vi "Destroy User Events.vi"(8 "error in (no error)":errorcluster, 11 "User Events Cluster_UI":T2) -> (0 "error out":errorcluster)   [LabVIEW 2019, in "ZenGage v3.0 UI.lvclass"]
uses:
  ZenGage v3.0 UI.lvclass
  Type Definitions/User Events UI/Optics diagnostics cluster.ctl
  <vilib>/vision/Image Controls.llb/IMAQ Image.ctl
  Type Definitions/Inspection/Result Cluster.ctl
  Type Definitions/User Events UI/LoadingBar_General_UI.ctl
  Common/Controls/Pop-up Input.ctl
  Type Definitions/JSON Read/Data initialization.ctl
  Type Definitions/JSON Read/Post select init.ctl
  Type Definitions/Diagnostics/Trigger sensor.ctl
  Type Definitions/User Events UI/UserEvents_UI.ctl
  Type Definitions/JSON Read/UI JSON read cluster.ctl
  Type Definitions/General/JSONRead.ctl
  Type Definitions/Inspection/Inspection Cluster.ctl
  Type Definitions/Diagnostics/Diagnostics(Cluster).ctl
  Type Definitions/Edit tolerance settings/Rack Selection.ctl
  <vilib>/Utility/miscctls.llb/LVPoint32TypeDef.ctl
  Type Definitions/Edit tolerance settings/Edit Tolerance Input.ctl
  Type Definitions/Edit tolerance settings/Edit Tolerance Overall Cluster.ctl
  Type Definitions/Controls and Indicators/Select a part (combobox).ctl
  Type Definitions/Controls and Indicators/EDL control references.ctl
  Type Definitions/Controls and Indicators/Diagnostics control referencs.ctl
  Type Definitions/Controls and Indicators/Inspection control references.ctl
  Type Definitions/Controls and Indicators/General_Control references.ctl
  Type Definitions/Controls and Indicators/Controls and Indicators Cluster.ctl
  Type Definitions/General/UI States(UI button enable disable).ctl
  Type Definitions/General/UIDataCluster.ctl
  Type Definitions/User Events UI/Stop slave cluster.ctl
  Type Definitions/General/Master sample references.ctl
panel:
  in  "Slave Loop":T1
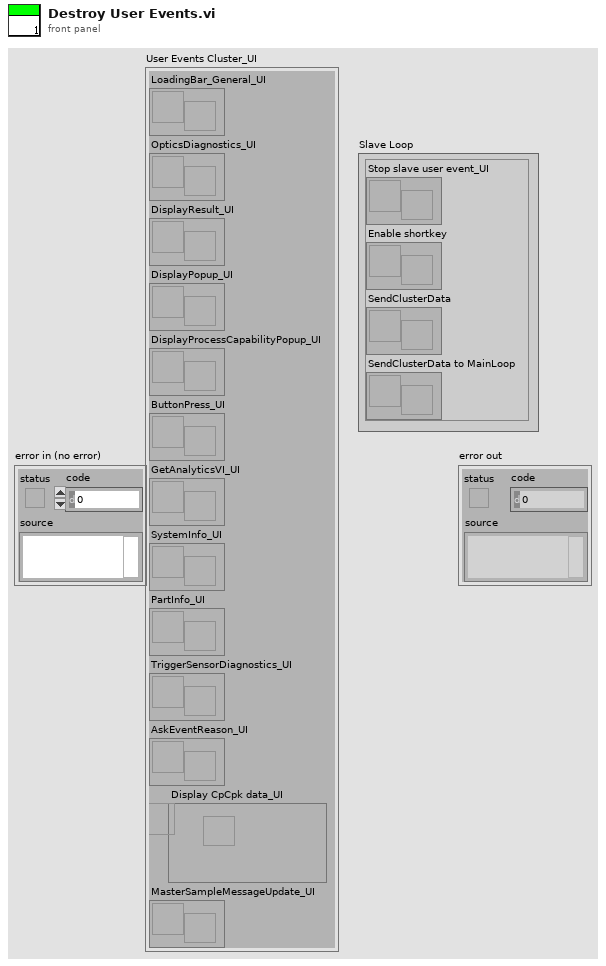
[diagram p1: front panel]
types:
  T1 = cluster{"Stop slave user event_UI":refnum<user-event>, "Enable shortkey":refnum<user-event>, "SendClusterData":refnum<user-event>, "SendClusterData to MainLoop":refnum<user-event>}
  T2 = typedef "ZenGage v3.0 UI.lvclass/UserEvents_UI.ctl" = cluster{"LoadingBar_General_UI":refnum<user-event>, "OpticsDiagnostics_UI":refnum<user-event>, "DisplayResult_UI":refnum<user-event>, "DisplayPopup_UI":refnum<user-event>, "DisplayProcessCapabilityPopup_UI":refnum<user-event>, "ButtonPress_UI":refnum<user-event>, "GetAnalyticsVI_UI":refnum<user-event>, "SystemInfo_UI":refnum<user-event>, "PartInfo_UI":refnum<user-event>, "TriggerSensorDiagnostics_UI":refnum<user-event>, "AskEventReason_UI":refnum<user-event>, "Display CpCpk data_UI":refnum<user-event>, "MasterSampleMessageUpdate_UI":refnum<user-event>}
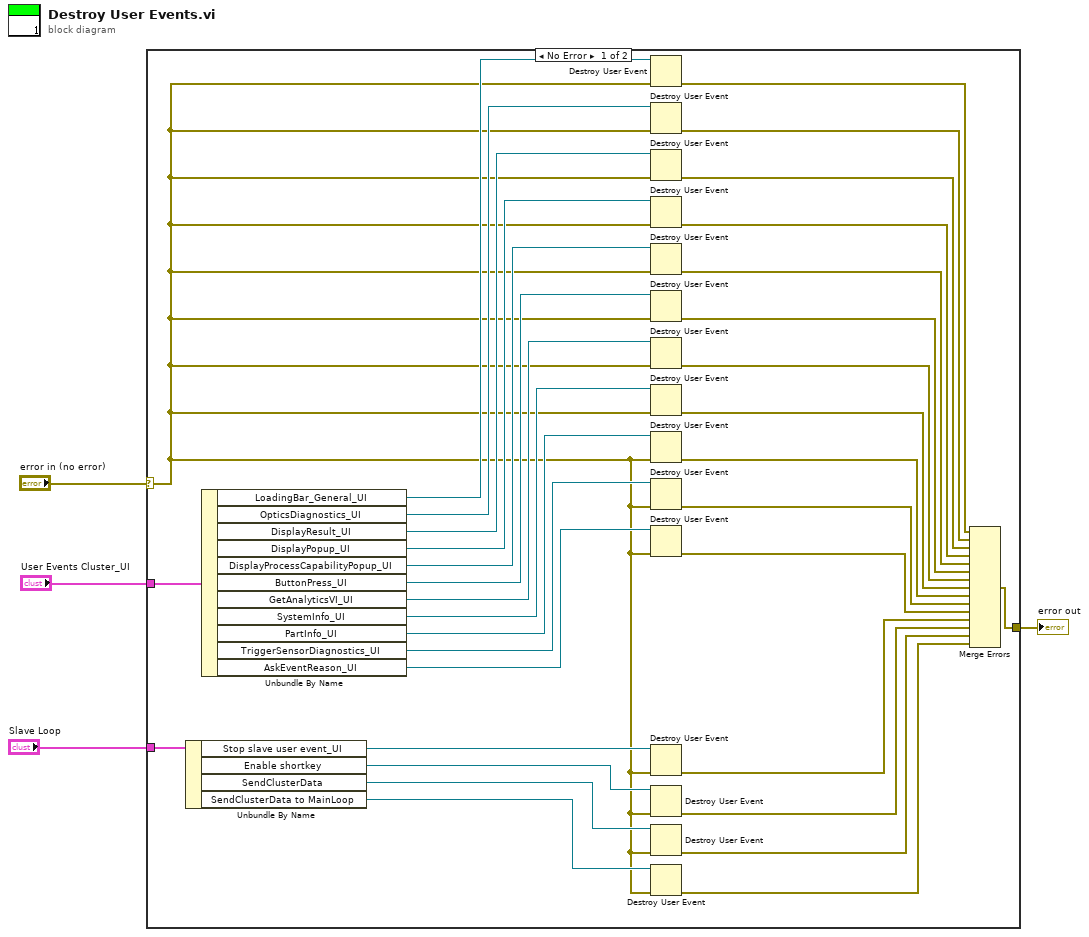
[diagram p0: block diagram]
diagram:
  n1 = case shown="No Error" "error in (no error)" {
    selector: "error in (no error)" -> [w9 w39]
    tunnel: [w25 w39] -> w3
    tunnel: "User Events Cluster_UI" -> [w15 _]
    tunnel: "Slave Loop" -> [w14 _]
    frame No Error {
      n2 = Unbundle By Name(w14) -> ("Stop slave user event_UI"=w13:refnum<user-event>, "Enable shortkey"=w12:refnum<user-event>, "SendClusterData"=w11:refnum<user-event>, "SendClusterData to MainLoop"=w10:refnum<user-event>)
      n3 = Unbundle By Name(w15) -> ("LoadingBar_General_UI"=w38:refnum<user-event>, "OpticsDiagnostics_UI"=w37:refnum<user-event>, "DisplayResult_UI"=w24:refnum<user-event>, "DisplayPopup_UI"=w23:refnum<user-event>, "DisplayProcessCapabilityPopup_UI"=w22:refnum<user-event>, "ButtonPress_UI"=w21:refnum<user-event>, "GetAnalyticsVI_UI"=w20:refnum<user-event>, "SystemInfo_UI"=w19:refnum<user-event>, "PartInfo_UI"=w18:refnum<user-event>, "TriggerSensorDiagnostics_UI"=w17:refnum<user-event>, "AskEventReason_UI"=w16:refnum<user-event>)
      n4 = Destroy User Event(user event=w38, error in=w9) -> (error out=w36:errorcluster)
      n5 = Destroy User Event(user event=w37, error in=w9) -> (error out=w35:errorcluster)
      n6 = Destroy User Event(user event=w24, error in=w9) -> (error out=w34:errorcluster)
      n7 = Destroy User Event(user event=w23, error in=w9) -> (error out=w33:errorcluster)
      n8 = Destroy User Event(user event=w22, error in=w9) -> (error out=w32:errorcluster)
      n9 = Destroy User Event(user event=w21, error in=w9) -> (error out=w31:errorcluster)
      n10 = Destroy User Event(user event=w20, error in=w9) -> (error out=w30:errorcluster)
      n11 = Destroy User Event(user event=w19, error in=w9) -> (error out=w29:errorcluster)
      n12 = Destroy User Event(user event=w18, error in=w9) -> (error out=w28:errorcluster)
      n13 = Destroy User Event(user event=w17, error in=w9) -> (error out=w27:errorcluster)
      n14 = Destroy User Event(user event=w16, error in=w9) -> (error out=w26:errorcluster)
      n15 = Destroy User Event(user event=w13, error in=w9) -> (error out=w8:errorcluster)
      n16 = Destroy User Event(user event=w12, error in=w9) -> (error out=w7:errorcluster)
      n17 = Destroy User Event(user event=w11, error in=w9) -> (error out=w6:errorcluster)
      n18 = Destroy User Event(user event=w10, error in=w9) -> (error out=w5:errorcluster)
      n19 = Merge Errors(w36, w35, w34, w33, w32, w31, w30, w29, w28, w27, w26, w8, w7, w6, w5) -> (w25:errorcluster)
    }
    frame Error {
    }
  }
  "error out" <- w3
